vi "Main.Package Parameters for Asynch VIs.vi"(10 "State Variables":T1={"Main App"={"Device Error"={"status"=FALSE, "code"=0, "source"=""}, "FPGA Session"=0, "Incoming Decimation"=0, "Outgoing Decimation"=0, "Process"=refnum}, "Protocol App"={"XNET Settings"={"Database"="", "Cluster"="", "Port"="", "Baud rate [Bd]"=0, "Termination"=0, "Incoming Rate"=0, "Outcoming Rate"=1, "Write Decimation"=1}, "Data"=[], "DTCs"=[], "Sim Addresses LUT"=variant, "Data Table LUT"=variant, "MonitorTool.Network"={"Address"=0, "Name"=0}, "Name"=""}} {"Protocol App"."MonitorTool.Network"."Name" format="%.0x"; "Protocol App"."Data"."Network"."Name" format="%.0x"; "Protocol App"."Data"."IncomingRefs"."Data Reference" format="%.0x"; "Protocol App"."Data"."OutgoingRefs"."Data Reference" format="%.0x"; "Protocol App"."XNET Settings"."Termination" items=["Off", "On"]}) -> (3 "Array":cluster{"VI":refnum<vi>, "Parameters":variant}[](array[cluster]))   [LabVIEW 2015, in "J1939 Addon Engine.lvlib"]
uses:
  J1939 Addon Engine.lvlib
  Types/Main.State Variables.ctl
  <vilib>/NI/NIVS Inline Async API/_VS Inline Async API/VS Inline Async API/VS Inline Async API.lvclass
  Types/Main.Settings.ctl
  Types/Protocol.App Settings.ctl
  Shared/Types/XNET Settings.ctl
  Types/Protocol.XNET Refs.ctl
  <vilib>/NI Veristand/Custom Device API/Block Data Reference.ctl
  <vilib>/NI Veristand/Custom Device API/Data Reference.ctl
  Shared/Types/Monitor Settings.ctl
  Types/Engine.DTC Settings.ctl
  Shared/Types/Compiled Simulated Settings.ctl
  Types/Engine.DTC FIFOs.ctl
  <vilib>/NI Veristand/Custom Device API/Custom Device API.lvlib
  Shared/J1939 Addon Shared.lvlib
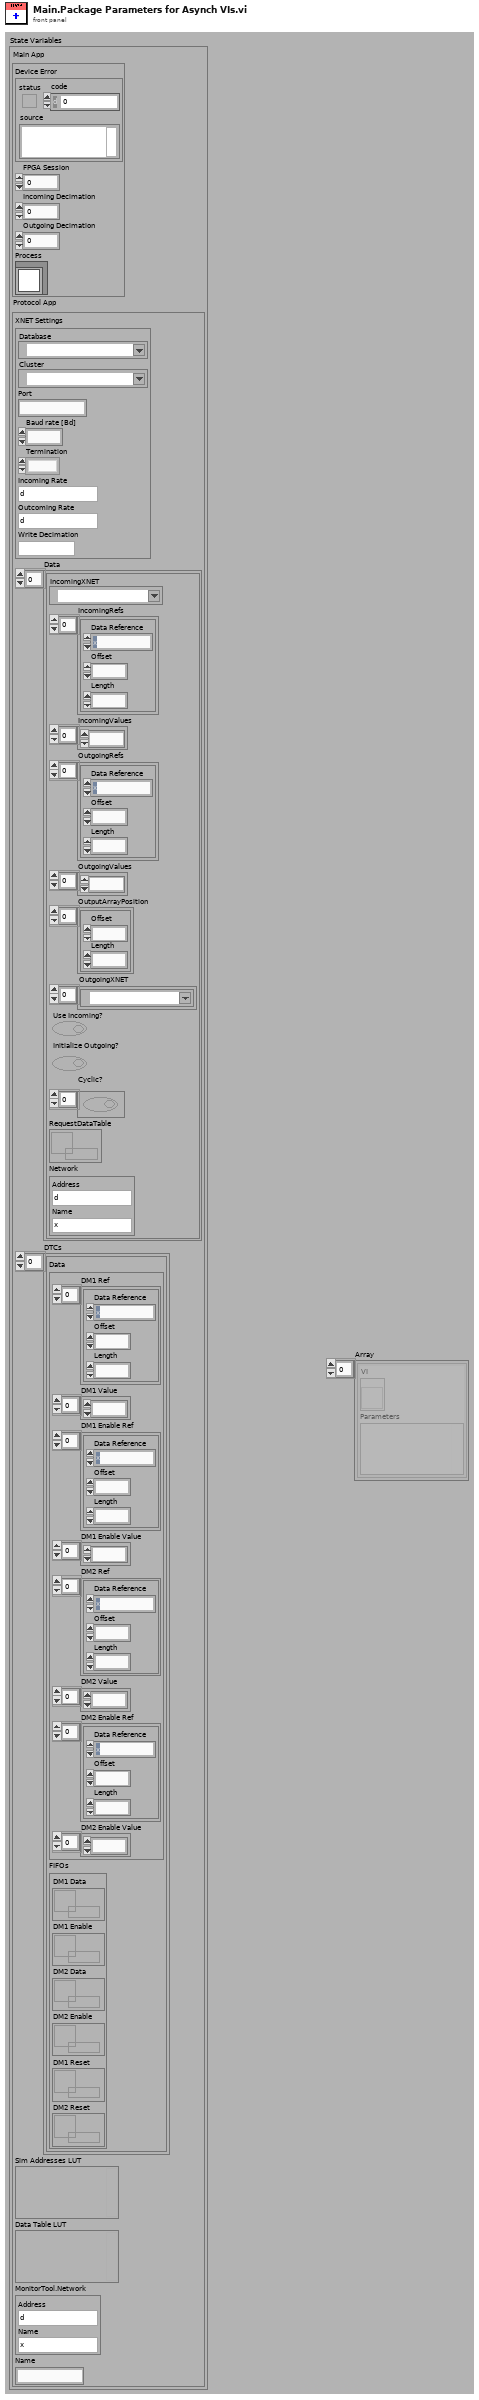
[diagram p1: front panel]
types:
  T1 = typedef "J1939 Addon Engine.lvlib/Main.State Variables.ctl" = cluster{"Main App":T2, "Protocol App":T3}
  T2 = typedef "J1939 Addon Engine.lvlib/Main.Settings.ctl" = cluster{"Device Error":errorcluster, "FPGA Session":u32, "Incoming Decimation":u32, "Outgoing Decimation":u32, "Process":refnum<class "VS Inline Async API.lvclass">}
  T3 = typedef "J1939 Addon Engine.lvlib/Protocol.App Settings.ctl" = cluster{"XNET Settings":T4, "Data":T5[], "DTCs":T9[], "Sim Addresses LUT":variant, "Data Table LUT":variant, "MonitorTool.Network":T8, "Name":string}
  T4 = typedef "J1939 Addon Shared.lvlib/XNET Settings.ctl" = cluster{"Database":refnum<k21>, "Cluster":refnum<k21>, "Port":string, "Baud rate [Bd]":u32, "Termination":u32, "Incoming Rate":u32, "Outcoming Rate":u32, "Write Decimation":u32}
  T5 = typedef "J1939 Addon Engine.lvlib/Protocol.XNET Refs.ctl" = cluster{"IncomingXNET":refnum<k21>, "IncomingRefs":T6[], "IncomingValues":dbl[], "OutgoingRefs":T6[], "OutgoingValues":dbl[], "OutputArrayPosition":cluster{"Offset":u32, "Length":u32}[], "OutgoingXNET":refnum<k21>[], "Use Incoming?":bool, "Initialize Outgoing?":bool, "Cyclic?":bool[], "RequestDataTable":refnum<k33>, "Network":T8}
  T6 = typedef "Custom Device API.lvlib/Block Data Reference.ctl" = cluster{"Data Reference":T7, "Offset":u64, "Length":u64}
  T7 = typedef "Custom Device API.lvlib/Data Reference.ctl" = i32
  T8 = typedef "J1939 Addon Shared.lvlib/Monitor Settings.ctl" = cluster{"Address":u8, "Name":u64}
  T9 = typedef "J1939 Addon Engine.lvlib/Engine.DTC Settings.ctl" = cluster{"Data":T10, "FIFOs":T11}
  T10 = typedef "J1939 Addon Shared.lvlib/Compiled Simulated Settings.ctl" = cluster{"DM1 Ref":T6[], "DM1 Value":dbl[], "DM1 Enable Ref":T6[], "DM1 Enable Value":dbl[], "DM2 Ref":T6[], "DM2 Value":dbl[], "DM2 Enable Ref":T6[], "DM2 Enable Value":dbl[]}
  T11 = typedef "J1939 Addon Engine.lvlib/Engine.DTC FIFOs.ctl" = cluster{"DM1 Data":refnum<k33>, "DM1 Enable":refnum<k33>, "DM2 Data":refnum<k33>, "DM2 Enable":refnum<k33>, "DM1 Reset":refnum<k33>, "DM2 Reset":refnum<k33>}
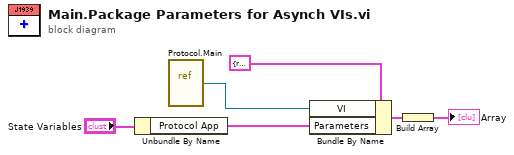
[diagram p0: block diagram]
diagram:
  n1 = Unbundle By Name("State Variables") -> ("Protocol App"=w5:T3)
  n2 = vi-ref "Protocol.Main.vi"() -> (w2:refnum<vi>)
  n3 = Bundle By Name(cluster=cluster{"VI":refnum<vi>, "Parameters":variant} {"VI"=refnum, "Parameters"=variant} ("Process"), "VI"=w2, "Parameters"=w5) -> (w3:cluster{"VI":refnum<vi>, "Parameters":variant})
  n4 = Build Array(w3) -> (→"Array":cluster{"VI":refnum<vi>, "Parameters":variant}[])
